vi "CheckMonthDateFolder_FarNearFieldREFS.vi"(0 "Folder Path Control":path, 1 "File Name":string, 3 "Overwrite?":bool, 4 "Automatic date folder nesting?":bool) -> (7 "File Path":path, 8 "Message":string, 9 "Warning":bool)   [LabVIEW 2014]
uses:
  <vilib>/regexp/Match Regular Expression.xnode
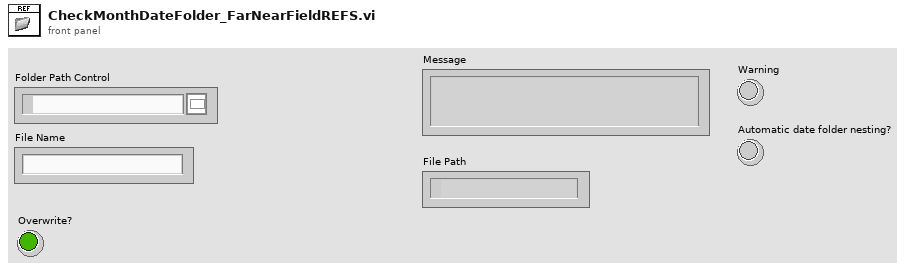
[diagram p1: front panel]
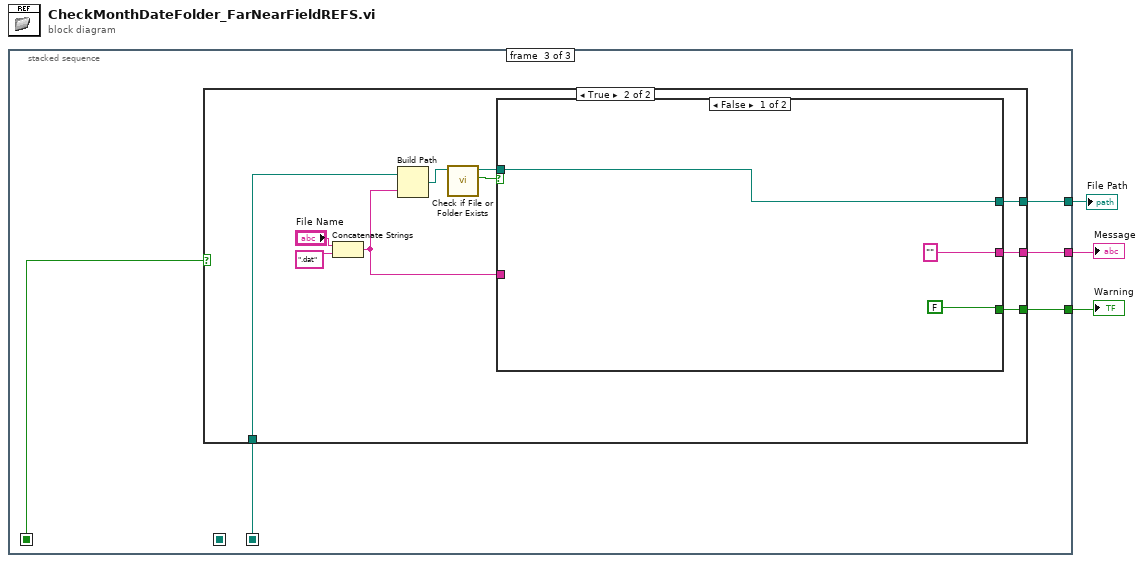
[diagram p0: block diagram]
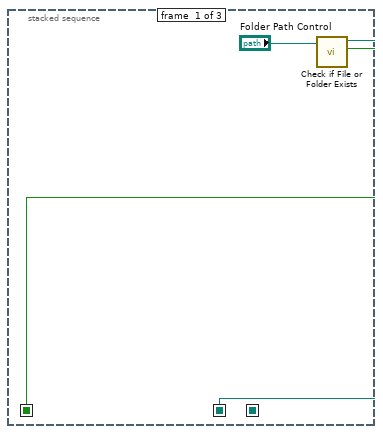
[diagram p2: hidden frame]
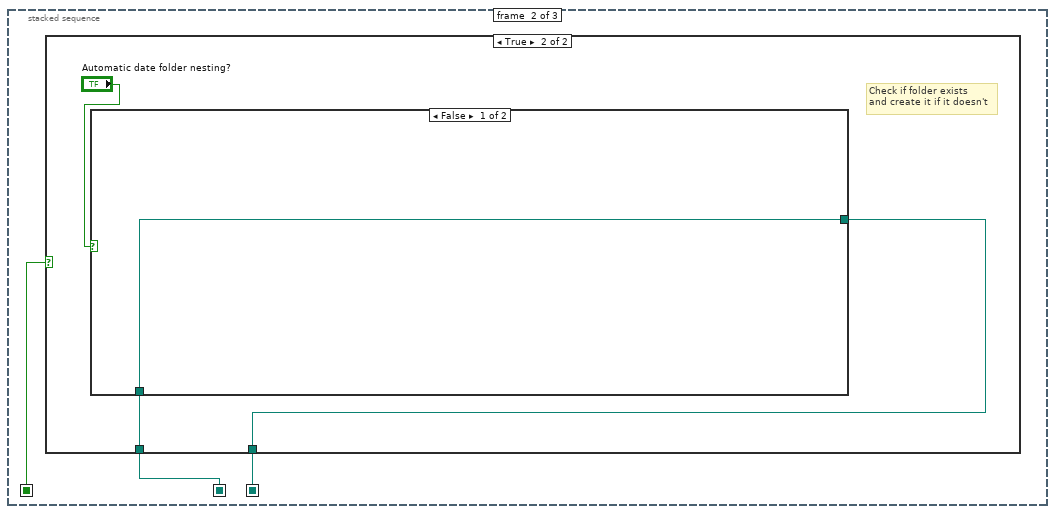
[diagram p3: hidden frame]
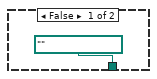
[diagram p4: hidden frame]
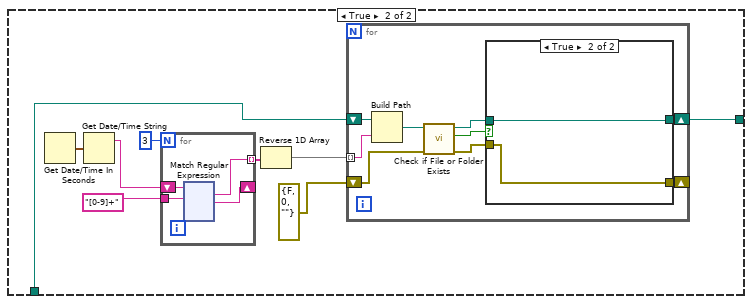
[diagram p5: hidden frame]
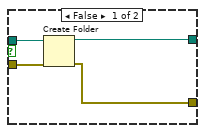
[diagram p6: hidden frame]
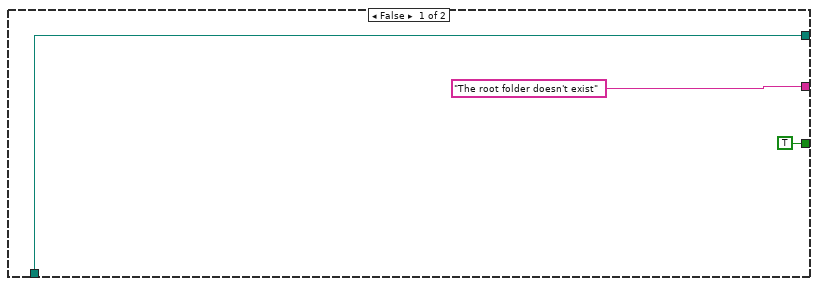
[diagram p7: hidden frame]
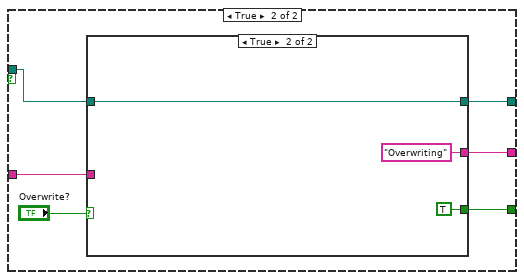
[diagram p8: hidden frame]
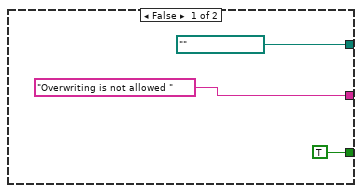
[diagram p9: hidden frame]
diagram:
  n1 = stacked-sequence {
    seq-local: [_ w9 _] -> [_ _ w161]
    seq-local: [w5 _ _] -> [_ w8 _]
    seq-local: [w4 _ _] -> [_ w7 w157]
    tunnel: [_ _ w160] -> w3
    tunnel: [_ _ w159] -> w2
    tunnel: [_ _ w158] -> w1
    frame #0 {
      n2 = call <vilib>:"Check if File or Folder Exists.vi"("path"="Folder Path Control") -> ("file or folder exists?"=w4:bool, "dup path"=w5:path)  [unwired: 8 in, 1 out]
    }
    frame #1 {
      n3 = case shown="True" w7 {
        tunnel: [path "" ("dup path") w13] -> w9
        tunnel: w8 -> [_ w12]
        frame False {
        }
        frame True {
          # "Check if folder exists\nand create it if it doesn't"
          n4 = case shown="False" "Automatic date folder nesting?" {
            tunnel: [w14 w16] -> w13
            tunnel: w12 -> [w14 w15]
            frame False {
            }
            frame True {
              n5 = Get Date/Time In Seconds() -> (seconds since 1Jan1904=w23:timestamp)
              n6 = Get Date/Time String(seconds (now)=w23) -> (date string=w22:string)  [unwired: 2 in, 1 out]
              n7 = for {
                N: 3 -> [_]
                tunnel: "[0-9]+" ("regular expression") -> [w41]
                tunnel: [w40] -> w19 mode=indexing
                shift-right: [w39] -> _
                shift-left: w22 -> [w42]
                n8 = xnode "Match Regular Expression"("input string"=w42, "regular expression"=w41) -> ("whole match"=w40:string, "after match"=w39:string)  [unwired: 4 in, 3 out]
              }
              n9 = Reverse 1D Array(array=w19) -> (reversed array=w18:string[])
              n10 = for {
                tunnel: w18 -> [w31] mode=indexing
                shift-right: [w25] -> w16
                shift-left: w15 -> [w32]
                shift-right: [w24] -> _
                shift-left: errorcluster {"status"=FALSE, "code"=0, "source"=""} ("error in (no error)") -> [w26]
                n11 = Build Path(base path=w32, name or relative path=w31) -> (appended path=w30:path)
                n12 = call <vilib>:"Check if File or Folder Exists.vi"("error in (no error)"=w26, "path"=w30) -> ("error out"=w27:errorcluster, "file or folder exists?"=w29:bool, "dup path"=w28:path)  [unwired: 7 in]
                n13 = case shown="True" w29 {
                  tunnel: w28 -> [w36 w38]
                  tunnel: w27 -> [w35 w37]
                  tunnel: [w34 w38] -> w25
                  tunnel: [w33 w37] -> w24
                  frame False {
                    n14 = Create Folder(path (use dialog)=w36, error in=w35) -> (created path=w34:path, error out=w33:errorcluster)  [unwired: 1 in, 1 out]
                  }
                  frame True {
                  }
                }
              }
            }
          }
        }
      }
    }
    frame #2 {
      n15 = case shown="True" w157 {
        tunnel: w161 -> [w164 w172]
        tunnel: [w164 w170] -> w160
        tunnel: [TRUE w169] -> w159
        tunnel: ["The root folder doesn't exist" w166] -> w158
        frame False {
        }
        frame True {
          n16 = Concatenate Strings("File Name", ".dat" ("string")) -> (w165:string)
          n17 = Build Path(base path=w172, name or relative path=w165) -> (appended path=w171:path)
          n18 = call <vilib>:"Check if File or Folder Exists.vi"("path"=w171) -> ("file or folder exists?"=w167:bool, "dup path"=w168:path)  [unwired: 8 in, 1 out]
          n19 = case shown="False" w167 {
            tunnel: [w177 w183] -> w170
            tunnel: [FALSE w182] -> w169
            tunnel: w168 -> [w177 w180]
            tunnel: ["" ("Message") w179] -> w166
            tunnel: w165 -> [_ w178]
            frame False {
            }
            frame True {
              n20 = case shown="True" "Overwrite?" {
                tunnel: [path "" ("File Path") w189] -> w183
                tunnel: [TRUE TRUE] -> w182
                tunnel: w180 -> [_ w189]
                tunnel: ["Overwriting is not allowed " ("Message") "Overwriting" ("Message")] -> w179
                tunnel: w178 -> [_ _]
                frame False {
                }
                frame True {
                }
              }
            }
          }
        }
      }
    }
  }
  "File Path" <- w3
  "Warning" <- w2
  "Message" <- w1
